vi "Cam-color5.vi"() -> ()   [LabVIEW 2018]
uses:
  <vilib>/vision/Classification.llb/IMAQ Classifier Session.ctl
  <vilib>/userdefined/High Color/IMAQdx.ctl
  <vilib>/vision/Classification.llb/IMAQ Classifier Read Options.ctl
  <vilib>/vision/NI_Vision_Development_Module.lvlib
  <vilib>/vision/driver/NI_Vision_Acquisition_Software.lvlib
panel:
  out "error out":errorcluster
  in  "error in 2":errorcluster
  out "Image":T1(plugin-control)
  in  "停止":bool
  out "error out 2":errorcluster
  out "Classes (Color Classification 1) 2":string[](array[string])
  out "Classifier Session (Color Classification 1) 2":T2
  out "Buffer Number Out":u32
  out "Processed Frames/s":dbl
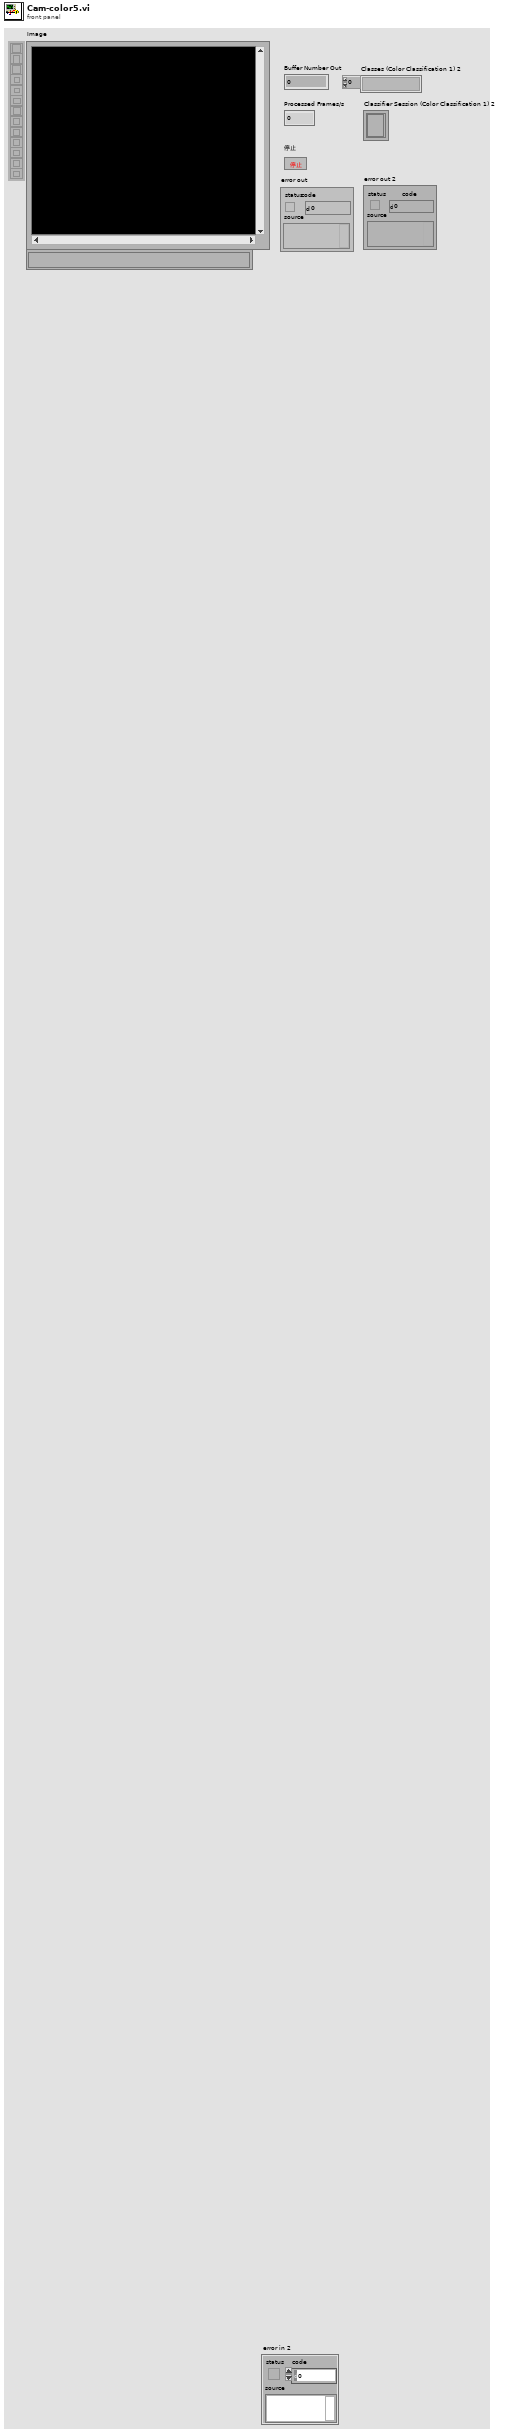
[diagram p1: front panel]
types:
  T1 = typedef "IMAQ Image.ctl" = refnum<image>
  T2 = typedef "IMAQ Classifier Session.ctl" = refnum<k1>
  T3 = typedef "IMAQdx.ctl" = refnum<k21>
  T4 = cluster{"Global Rectangle":i32[], "Contours":cluster{"ID":enum32{"External", "Internal"}, "Type":u32, "Coordinates":i32[]}[]}
  T5 = typedef "IMAQ Classifier Read Options.ctl" = i32
  T6 = typedef "ROI Descriptor" = cluster{"Global Rectangle":i32[], "Contours":cluster{"ID":enum32{"External", "Internal"}, "Type":u32, "Coordinates":i32[]}[]}
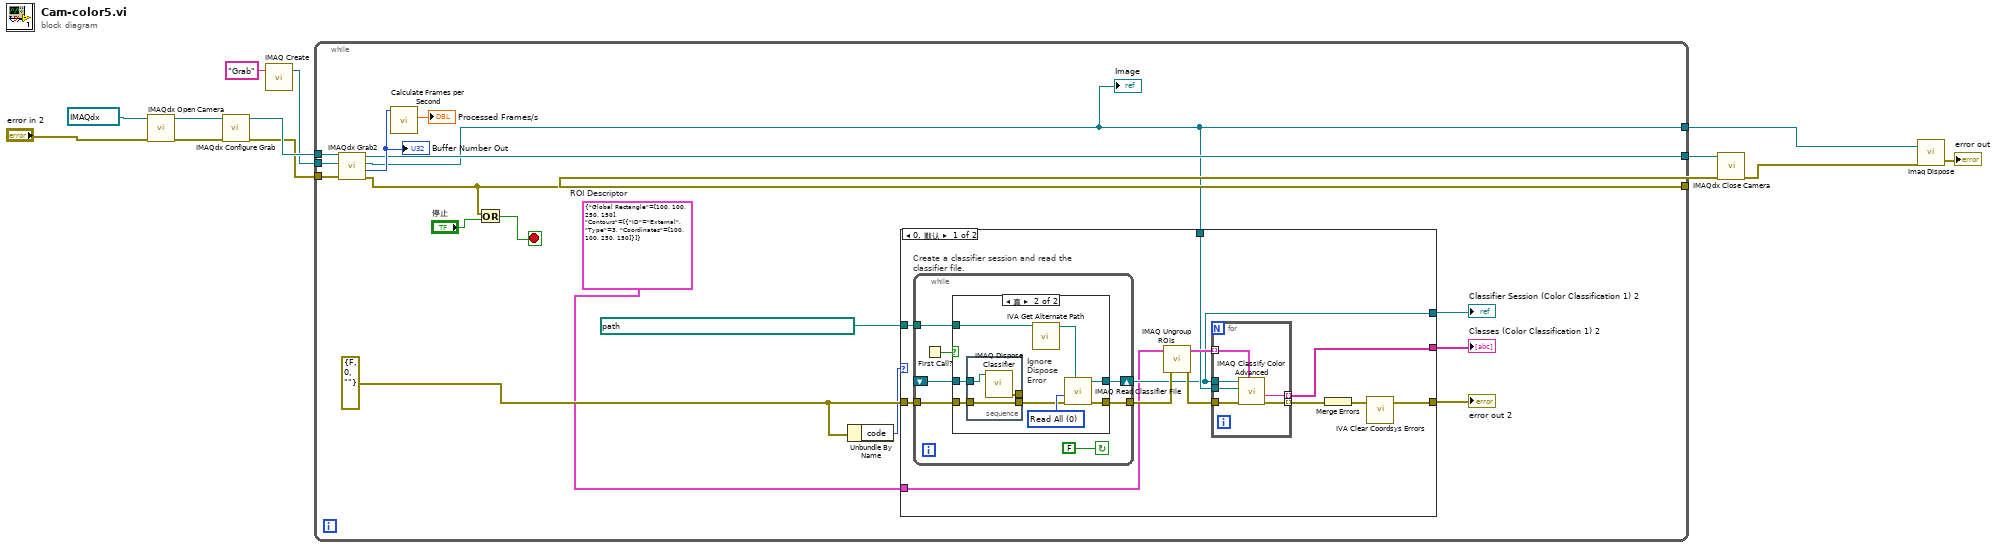
[diagram p0: block diagram]
diagram:
  n1 = call <vilib>:"IMAQdx Open Camera.vi"("error in"="error in 2", "Session In"=T3 "cam1") -> ("error out"=w11:errorcluster, "Session Out"=w13:T3)  [unwired: 8 in]
  n2 = call <vilib>:"IMAQdx Configure Grab.vi"("error in"=w11, "Session In"=w13) -> ("error out"=w3:errorcluster, "Session Out"=w12:T3)  [unwired: 8 in]
  n3 = call "IMAQ Create"("Image Name"="Grab") -> ("New Image"=w10:T1)  [unwired: 4 in, 1 out]
  n4 = while {
    tunnel: w12 -> [w30]
    tunnel: w10 -> [w29]
    tunnel: [w14] -> w7
    tunnel: [w24] -> w6
    tunnel: [w26] -> w5
    tunnel: w3 -> [w25]
    stop <- w16 stop-if-true
    w15 = T4 {"Global Rectangle"=[100, 100, 250, 150], "Contours"=[{"ID"=enum."External", "Type"=3, "Coordinates"=[100, 100, 250, 150]}]}  # ROI Descriptor
    w19 = errorcluster {"status"=FALSE, "code"=0, "source"=""} ("error in 2")
    n5 = call <vilib>:"IMAQdx Grab2.vi"("error in"=w25, "Image In"=w29, "Session In"=w30) -> ("error out"=w24:errorcluster, "Buffer Number Out"=w28:u32, "Image Out"=w14:T1, "Session Out"=w26:T3)  [unwired: 5 in]
    "Buffer Number Out" <- w28
    "Image" <- w14
    n6 = call <vilib>:"Calculate Frames per Second.vi"("Buffer Number"=w28) -> ("Processed Frames/s"=→"Processed Frames/s":dbl)  [unwired: 8 in, 2 out]
    n7 = Or(x=w24, y="停止") -> (x .or. y?=w16:bool)
    n8 = Unbundle By Name(w19) -> ("code"=w18:i32)
    n9 = case shown="0, 默认" w18 {
      tunnel: [w32 _] -> w23
      tunnel: [w42 _] -> w22
      tunnel: [w36 _] -> w21
      tunnel: path "D:/Labviewprogram/视觉/视觉框架/Color 识别.clf" ("File Path") -> [w35 _]
      tunnel: w19 -> [w34 _]
      tunnel: w14 -> [w33 _]
      tunnel: w15 -> [w31 _]
      frame 0, Default {
        n10 = while "Create a classifier session and read the classifier file." {
          shift-right: [w55] -> w32
          shift-left: _ -> [w54]
          tunnel: w34 -> [w52]
          tunnel: [w51] -> w37
          tunnel: w35 -> [w50]
          stop <- FALSE continue-if-true
          n11 = First Call?() -> (First Call?: T/F=w49:bool)
          n12 = case "条件结构" shown="真" w49 {
            tunnel: [w57 w64] -> w55
            tunnel: w54 -> [w57 w62]
            tunnel: w52 -> [w56 w61]
            tunnel: [w56 w63] -> w51
            tunnel: w50 -> [_ w59]
            frame False {
            }
            frame True {
              w65 = T5 0 items=["Read All", "Add Samples, Do Not Change Options", "Read Options, Do Not Add Samples"] ("Read Options")
              # "Ignore Dispose Error"
              n13 = stacked-sequence "层叠式顺序结构" {
                tunnel: w62 -> [w68]
                tunnel: w61 -> [w67]
                tunnel: [w67] -> w60
                tunnel: [w66] -> _
                frame #0 {
                  n14 = call "IMAQ Dispose Classifier"("Classifier Session"=w68) -> ("error out"=w66:errorcluster)  [unwired: 1 in, 9 out]
                }
              }
              n15 = call <vilib>:"IVA Get Alternate Path.vi"("Path In"=w59) -> ("Path Out"=w58:path)  [unwired: 10 out]
              n16 = call "IMAQ Read Classifier File"("File Path"=w58, "error in (no error)"=w60, "Read Options"=w65) -> ("error out"=w63:errorcluster, "Classifier Session"=w64:T2)  [unwired: 1 in, 6 out]
            }
          }
        }
        n17 = call "IMAQ Ungroup ROIs"("error in (no error)"=w37, "ROI Descriptor"=w31) -> ("error out"=w38:errorcluster, "ROI Descriptors out"=w39:T6[])  [unwired: 2 out]
        n18 = for "For循环" {
          tunnel: [w48] -> w36 mode=indexing
          tunnel: [w47] -> w40 mode=indexing
          tunnel: w38 -> [w45]
          tunnel: w39 -> [w44] mode=indexing
          tunnel: w33 -> [w43]
          tunnel: w32 -> [w46]
          n19 = call "IMAQ Classify Color Advanced"("ROI Descriptor"=w44, "error in (no error)"=w45, "Image"=w43, "Classifier Session"=w46) -> ("error out"=w47:errorcluster, "Class"=w48:string)  [unwired: 6 out]
        }
        n20 = Merge Errors(w40) -> (w41:errorcluster)
        n21 = call <vilib>:"IVA Clear Coordsys Errors.vi"("error in (no error)"=w41) -> ("error out"=w42:errorcluster)  [unwired: 10 in]
      }
      frame 1 {
      }
    }
    "error out 2" <- w22
    "Classes (Color Classification 1) 2" <- w21
    "Classifier Session (Color Classification 1) 2" <- w23
  }
  n22 = call <vilib>:"IMAQdx Close Camera.vi"("error in"=w6, "Session In"=w5) -> ("error out"=w4:errorcluster)  [unwired: 9 in]
  n23 = call "Imaq Dispose"("Image"=w7, "error in (no error)"=w4) -> ("error out"=→"error out":errorcluster)  [unwired: 4 in]
